vi "Plug_in_Directories.vi"() -> (0 "Final":path, 1 "Per Block":path, 2 "Pre_Analysis_Analogue_Plugins":path, 3 "Initial":path)   [LabVIEW 2011]
uses:
  Globals/Constants_global.vi
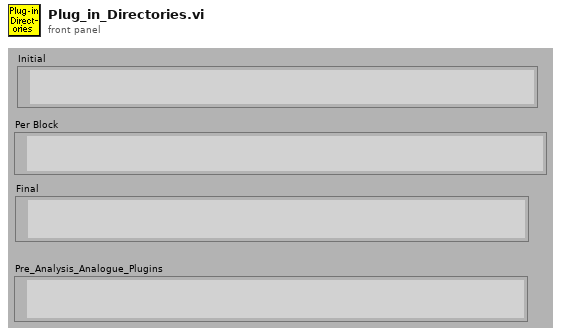
[diagram p1: front panel]
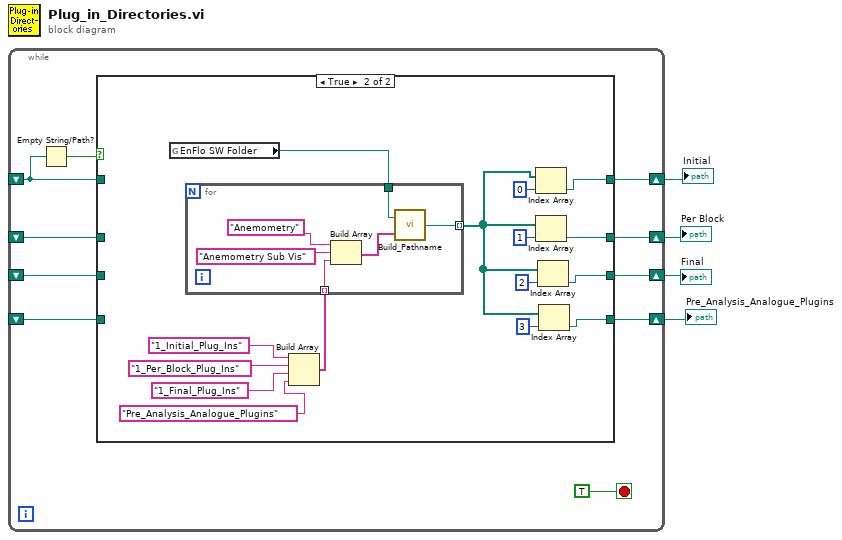
[diagram p0: block diagram]
diagram:
  n1 = while {
    shift-right: [w12] -> w2
    shift-left: _ -> [w9]
    shift-right: [w11] -> w3
    shift-left: _ -> [w8]
    shift-right: [w10] -> w4
    shift-left: _ -> [w7]
    shift-right: [w6] -> w1
    shift-left: _ -> [w5]
    stop <- TRUE stop-if-true
    n2 = Empty String/Path?(string/path=w9) -> (empty?=w13:bool)
    n3 = case shown="True" w13 {
      tunnel: [w18 w25] -> w12
      tunnel: [w17 w24] -> w11
      tunnel: [w16 w23] -> w10
      tunnel: w9 -> [w18 _]
      tunnel: w8 -> [w17 _]
      tunnel: w7 -> [w16 _]
      tunnel: [w15 w21] -> w6
      tunnel: w5 -> [w15 _]
      frame False {
      }
      frame True {
        n4 = global read "Constants_global.vi" "EnFlo SW Folder"() -> (w30:path)
        n5 = Build Array("1_Initial_Plug_Ins", "1_Per_Block_Plug_Ins", "1_Final_Plug_Ins", "Pre_Analysis_Analogue_Plugins") -> (w29:string[])
        n6 = for {
          tunnel: w30 -> [w36]
          tunnel: w29 -> [w35] mode=indexing
          tunnel: [w34] -> w19 mode=indexing
          n7 = Build Array("Anemometry", "Anemometry Sub Vis", w35) -> (w39:string[])
          n8 = call "Build_Pathname.vi"("PathElements"=w39, "PathnameIn"=w36) -> ("AppendedPath"=w34:path)
        }
        n9 = Index Array(array=w19, index=0) -> (element=w25:path)
        n10 = Index Array(array=w19, index=1) -> (element=w24:path)
        n11 = Index Array(array=w19, index=2) -> (element=w23:path)
        n12 = Index Array(array=w19, index=3) -> (element=w21:path)
      }
    }
  }
  "Initial" <- w2
  "Final" <- w4
  "Per Block" <- w3
  "Pre_Analysis_Analogue_Plugins" <- w1
